vi "Align & Distribute UI.vi"() -> (0 "Distribute Type valid?":bool, 1 "Align Type valid?":bool, 2 "Distribute Type":T11(ring), 3 "Align Type":T12(ring))   [LabVIEW 2020, in "Align and Distribute.lvlib"]
uses:
  Align and Distribute.lvlib
  Align Objects.ctl
  Distribute Objects.ctl
  Dist Top Edges.ctl
  Dist Bottom Edges.ctl
  Dist Vertical Gap.ctl
  Dist Vertical Compress.ctl
  Dist Left Edges.ctl
  Dist Horizontal Centers.ctl
  Dist Right Edges.ctl
  Dist Horizontal Gap.ctl
  Dist Horizontal Compress.ctl
panel:
  out "Label":string
  in  "Distribute Objects":T1
  in  "Align Objects":T13
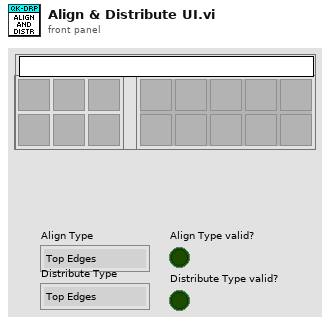
[diagram p1: front panel]
types:
  T1 = typedef "Align and Distribute.lvlib/Distribute Objects.ctl" = cluster{"Top Edges":T2, "Vertical Centers":bool, "Bottom Edges":T3, "Vertical Gap":T4, "Vertical Compress":T5, "Left Edges":T6, "Horizontal Centers":T7, "Right Edges":T8, "Horizontal Gap":T9, "Horizontal Compress":T10}
  T2 = typedef "Align and Distribute.lvlib/Dist Top Edges.ctl" = bool
  T3 = typedef "Align and Distribute.lvlib/Dist Bottom Edges.ctl" = bool
  T4 = typedef "Align and Distribute.lvlib/Dist Vertical Gap.ctl" = bool
  T5 = typedef "Align and Distribute.lvlib/Dist Vertical Compress.ctl" = bool
  T6 = typedef "Align and Distribute.lvlib/Dist Left Edges.ctl" = bool
  T7 = typedef "Align and Distribute.lvlib/Dist Horizontal Centers.ctl" = bool
  T8 = typedef "Align and Distribute.lvlib/Dist Right Edges.ctl" = bool
  T9 = typedef "Align and Distribute.lvlib/Dist Horizontal Gap.ctl" = bool
  T10 = typedef "Align and Distribute.lvlib/Dist Horizontal Compress.ctl" = bool
  T11 = enum32{"Top Edges", "Vertical Centers", "Bottom Edges", "Vertical Gap", "Vertical Compress", "Left Edges", "Horizontal Centers", "Right Edges", "Horizontal Gap", "Horizontal Compress"}
  T12 = enum32{"Top Edges", "Vertical Centers", "Bottom Edges", "Left Edges", "Horizontal Centers", "Right Edges"}
  T13 = typedef "Align and Distribute.lvlib/Align Objects.ctl" = cluster{"Top Edges":bool, "Vertical Centers":bool, "Bottom Edges":bool, "Left Edges":bool, "Horizontal Centers":bool, "Right Edges":bool}
  T14 = typedef "eventvkey.ctl" = enum16{"ASCII", "Enter", "Return", "Shift", "Ctrl", "Alt", "Cmd", "Opt", "Caps", "NumLock", "Clear", "Break", "Up", "Down", "Left", "Right", "Insert", "Delete", "Home", "End", "PageUp", "PageDown", "Escape", "Help", "Pause", "ScrollLock", "F1", "F2", "F3", "F4", "F5", "F6", "F7", "F8", "F9", "F10", "F11", "F12", "F13", "F14", "F15", "F16", "F17", "F18", "F19", "F20", "F21", "F22", "F23", "F24", "Play", "VolumeUp", "VolumeDown", "Mute", "Two Byte Char"}
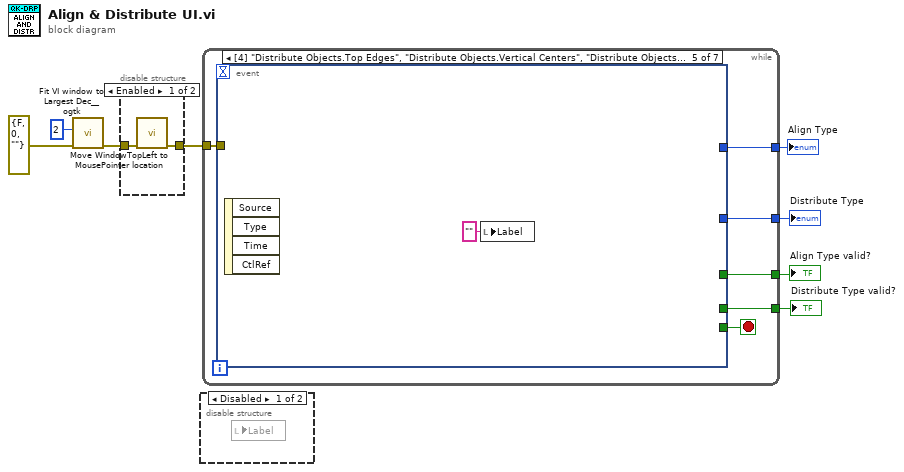
[diagram p0: block diagram]
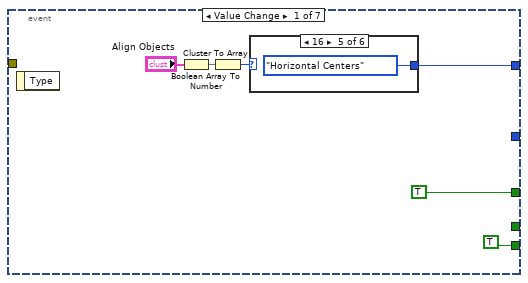
[diagram p4: hidden frame]
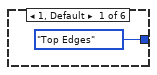
[diagram p5: hidden frame]
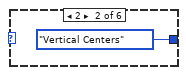
[diagram p6: hidden frame]
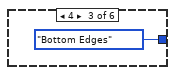
[diagram p7: hidden frame]
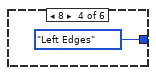
[diagram p8: hidden frame]
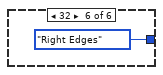
[diagram p9: hidden frame]
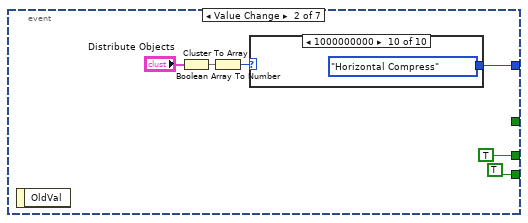
[diagram p10: hidden frame]
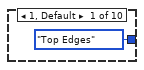
[diagram p11: hidden frame]
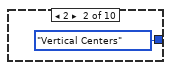
[diagram p12: hidden frame]
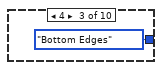
[diagram p13: hidden frame]
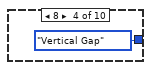
[diagram p14: hidden frame]
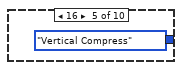
[diagram p15: hidden frame]
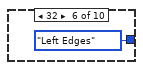
[diagram p16: hidden frame]
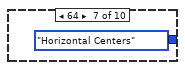
[diagram p17: hidden frame]
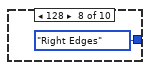
[diagram p18: hidden frame]
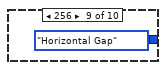
[diagram p19: hidden frame]
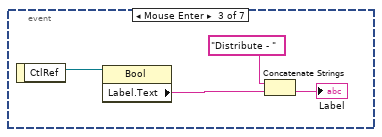
[diagram p20: hidden frame]
diagram:
  n1 = call <userlib>:"Fit VI window to Largest Dec__ogtk.vi"("error in (no error)"=errorcluster {"status"=FALSE, "code"=0, "source"=""}, "border spacing (2 px)"=2) -> ("error out"=w1:errorcluster)  [unwired: 4 in, 1 out]
  n2 = disable-structure shown="Enabled" {
    disable-tunnel: [w10 w11] -> w6
    disable-tunnel: w1 -> [w9 w11]
    frame Enabled {
      n3 = call "Move WindowTopLeft to MousePointer location.vi"("error in (no error)"=w9) -> ("error out"=w10:errorcluster)  [unwired: 10 in]
    }
    frame Disabled {
    }
  }
  n4 = disable-structure shown="Disabled" {
    frame Disabled {
      n5 = local read "Label"() -> ()  [unwired: 1 in]
    }
    frame Enabled {
    }
  }
  n6 = while {
    tunnel: [w17] -> w8
    tunnel: [w16] -> w7
    tunnel: w6 -> [w15]
    tunnel: [w14] -> w5
    tunnel: [w13] -> w4
    stop <- w12 stop-if-true
    n7 = event shown="[4] \"Distribute Objects.Top Edges\", \"Distribute Objects.Vertical Centers\", \"Distribute Objects.Bottom Edges\", \"Distribute Objects.Vertical Gap\", \"Distribute Objects.Vertical Compress\", \"Distribute Objects.Left Edges\", \"Distribute Objects.Horizontal Centers\", \"Distribute Objects.Right Edges\", \"Distribute Objects.Horizontal Gap\", \"Distribute Objects.Horizontal Compress\": Mouse Leave" {
      selector: _ -> [_ _ _ _ _ _ _]
      dyn-events: _ -> [_ _ _ _ _ _ _]
      timeout: _ -> [_ _ _ _ _ _ _]
      tunnel: [w20 _ _ _ _ _ w62] -> w17
      tunnel: [_ w32 _ _ _ _ w61] -> w16
      tunnel: w15 -> [_ _ _ _ _ _ _]
      tunnel: [TRUE _ _ _ _ _ w58] -> w14
      tunnel: [_ TRUE _ _ _ _ w57] -> w13
      tunnel: [TRUE TRUE _ _ _ _ w56] -> w12
      event Value Change {
        n8 = event-data() -> ()  [unwired: 1 in, 1 out]
        n9 = Cluster To Array(cluster="Align Objects") -> (array=w22:bool[])
        n10 = Boolean Array To Number(Boolean array=w22) -> (number=w21:u32)
        n11 = case shown="16" w21 {
          tunnel: [T12."Top Edges" ("Align Type") T12."Vertical Centers" ("Align Type") T12."Bottom Edges" ("Align Type") T12."Left Edges" ("Align Type") T12."Horizontal Centers" ("Align Type") T12."Right Edges" ("Align Type")] -> w20
          frame 1, Default {
          }
          frame 2 {
          }
          frame 4 {
          }
          frame 8 {
          }
          frame 16 {
          }
          frame 32 {
          }
        }
      }
      event Value Change {
        n12 = event-data() -> ()  [unwired: 1 in, 1 out]
        n13 = Cluster To Array(cluster="Distribute Objects") -> (array=w33:T10[])
        n14 = Boolean Array To Number(Boolean array=w33) -> (number=w34:u32)
        n15 = case shown="1000000000" w34 {
          tunnel: [T11."Top Edges" ("DistributeType") T11."Vertical Centers" ("DistributeType") T11."Bottom Edges" ("DistributeType") T11."Vertical Gap" ("DistributeType") T11."Vertical Compress" ("DistributeType") T11."Left Edges" ("DistributeType") T11."Horizontal Centers" ("DistributeType") T11."Right Edges" ("DistributeType") T11."Horizontal Gap" ("DistributeType") T11."Horizontal Compress" ("DistributeType")] -> w32
          frame 1, Default {
          }
          frame 2 {
          }
          frame 4 {
          }
          frame 8 {
          }
          frame 16 {
          }
          frame 32 {
          }
          frame 64 {
          }
          frame 128 {
          }
          frame 256 {
          }
          frame 512 {
          }
        }
      }
      event Mouse Enter {
        n16 = event-data() -> ("CtlRef"=w49:refnum<vi>)  [unwired: 1 in]
        n17 = property class="Bool"(reference=w49) -> ("Label.Text"=w48:string)  [unwired: 1 in, 2 out]
        n18 = Concatenate Strings("Distribute - " ("string"), w48) -> (→"Label":string)
      }
      event Mouse Leave {
        n19 = event-data() -> ()  [unwired: 1 in, 1 out]
        n20 = local write "Label"("" ("Label")) -> ()
      }
      event Mouse Leave {
        n21 = event-data() -> ()  [unwired: 1 in, 4 out]
        n22 = local write "Label"("" ("Label")) -> ()
      }
      event Mouse Enter {
        n23 = event-data() -> ("CtlRef"=w55:refnum<vi>)  [unwired: 1 in]
        n24 = property class="Bool"(reference=w55) -> ("Label.Text"=w54:string)  [unwired: 1 in, 2 out]
        n25 = Concatenate Strings("Align - " ("string"), w54) -> (w52:string)
        n26 = local write "Label"(w52) -> ()
      }
      event Key Down {
        n27 = event-data() -> ("Char"=w63:i16, "VKey"=w59:T14)  [unwired: 1 in]
        n28 = To Unsigned Byte Integer(number=w63) -> (unsigned 8bit integer=w64:u8)
        n29 = Build Array(w64) -> (w65:u8[])
        n30 = Byte Array To String(unsigned byte array=w65) -> (string=w60:string)
        n31 = case shown="\"Escape\"" w59 {
          tunnel: [w70 _] -> w62
          tunnel: [w69 _] -> w61
          tunnel: w60 -> [w68 _]
          tunnel: [FALSE _] -> w58
          tunnel: [FALSE _] -> w57
          tunnel: [_ TRUE] -> w56
          frame "ASCII", Default {
            n32 = case shown="\"L\", \"l\", Default" w68 {
              tunnel: [T11."Vertical Compress" ("DistributeType") T11."Vertical Compress" ("DistributeType") T11."Horizontal Compress" ("DistributeType") T11."Horizontal Compress" ("DistributeType") T11."Horizontal Compress" ("DistributeType") T11."Vertical Compress" ("DistributeType")] -> w69
              frame "R", "r" {
              }
              frame "L", "l", Default {
              }
              frame "T", "t" {
              }
              frame "B", "b" {
              }
              frame "V", "v" {
              }
              frame "H", "h" {
              }
            }
            n33 = case shown="\"V\", \"v\"" w68 {
              tunnel: [T12."Right Edges" ("Align Type") T12."Left Edges" ("Align Type") T12."Top Edges" ("Align Type") T12."Bottom Edges" ("Align Type") T12."Vertical Centers" ("Align Type") T12."Horizontal Centers" ("Align Type")] -> w70
              frame "R", "r" {
              }
              frame "L", "l", Default {
              }
              frame "T", "t" {
              }
              frame "B", "b" {
              }
              frame "V", "v" {
              }
              frame "H", "h" {
              }
            }
          }
          frame "Escape" {
          }
        }
      }
    }
  }
  "Align Type" <- w8
  "Distribute Type" <- w7
  "Align Type valid?" <- w5
  "Distribute Type valid?" <- w4
